vi "GCSArray_header_read.vi"(0 "GCSArray input string":string, 1 "Range":T2, 5 "error in (no error)":errorcluster) -> (14 "GCSArray Header":T1={"Identifier"="", "Version"=0, "Remark"="", "Dimension"=0, "Type"=enum."Matrix", "Separator"=0, "NData"=0, "NData%"=[], "Name%"=[], "Start%"=[], "End%"=[], "Delta%"=[], "SampleTime"=inf, "TransmittedUnit%"=[], "DisplayedUnit%"=[], "RatioNominator%"=[], "RatioDenominator%"=[]}, 19 "error out":errorcluster)   [LabVIEW 2026]
doc: "Transforms an Input string, limited to a specific character Range, into a GCSArray header.\n\nThe conversion of the textual representation of a GCSArray into the native format is performed using the LabVIEW regular expression engine. In case a header entry is not found its value is set to the default value, which is usually zero. The implemented functionality uses the GCS Array Data Format Description (Release 1.2.1, Date: 2010-09-27, PI document code: SM146E)."
uses:
  GCSArray_regex_range.ctl
  GCSArray_header.ctl
  GCSArray_header_action.ctl
  GCSArray_regex_selector.ctl
panel:
  in  "GCSArray_header":T1={"Identifier"="", "Version"=0, "Remark"="", "Dimension"=0, "Type"=enum."Matrix", "Separator"=0, "NData"=0, "NData%"=[], "Name%"=[], "Start%"=[], "End%"=[], "Delta%"=[], "SampleTime"=inf, "TransmittedUnit%"=[], "DisplayedUnit%"=[], "RatioNominator%"=[], "RatioDenominator%"=[]}
  # "Read a GCS Array string from, extract the header informations\naccording to the GCSArray definitions and return the\ncorresponding 'GCSArray Header' object."
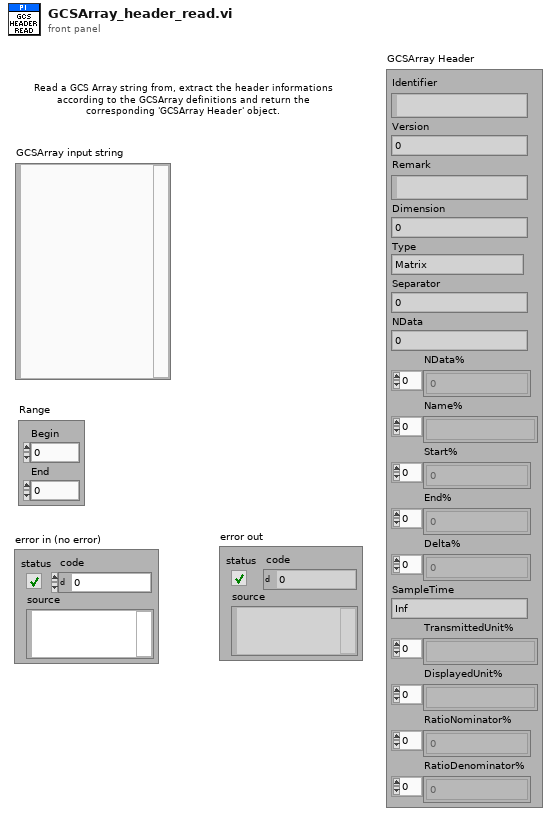
[diagram p1: front panel]
types:
  T1 = typedef "GCSArray_header.ctl" = cluster{"Identifier":string, "Version":i32, "Remark":string, "Dimension":i32, "Type":enum16{"Matrix", "Table"}, "Separator":u8, "NData":i32, "NData%":i32[], "Name%":string[], "Start%":dbl[], "End%":dbl[], "Delta%":dbl[], "SampleTime":dbl, "TransmittedUnit%":string[], "DisplayedUnit%":string[], "RatioNominator%":dbl[], "RatioDenominator%":dbl[]}
  T2 = typedef "GCSArray_regex_range.ctl" = cluster{"Begin":i32, "End":i32}
  T3 = typedef "GCSArray_regex_selector.ctl" = enum16{"GCS_ARRAY Block Full", "GCS_ARRAY Block ID", "GCS_ARRAY Block Header", "GCS_ARRAY Block Data", "GCS_ARRAY Identifier", "GCS_ARRAY Remark", "GCS_ARRAY Version", "GCS_ARRAY Dimension", "GCS_ARRAY Type", "GCS_ARRAY Separator", "GCS_ARRAY NData", "GCS_ARRAY NData%", "GCS_ARRAY NData% Keyword", "GCS_ARRAY Name%", "GCS_ARRAY Name% Keyword", "GCS_ARRAY Start%", "GCS_ARRAY Start% Keyword", "GCS_ARRAY End%", "GCS_ARRAY End% Keyword", "GCS_ARRAY Delta%", "GCS_ARRAY Delta% Keword", "GCS_ARRAY Sample Time", "GCS_ARRAY Unit of transmitted value%", "GCS_ARRAY Trans_Unit% Keyword", "GCS_ARRAY Trans_Unit% = RAW Keyword", "GCS_ARRAY Unit of displayed value%", "GCS_ARRAY Disp_Unit% Keyword", "GCS_ARRAY Nominator%", "GCS_ARRAY Ratio_Nom% Keyword", "GCS_ARRAY Denominator%", "GCS_ARRAY Ratio_Denom% Keyword", "GCS_ARRAY End of Header", "GCS_ARRAY Empty line of Header"}
  T4 = typedef "GCSArray_header_action.ctl" = enum16{"GCS_ARRAY_HEADER Identifier", "GCS_ARRAY_HEADER Version", "GCS_ARRAY_HEADER Remark", "GCS_ARRAY_HEADER Dimension", "GCS_ARRAY_HEADER Type", "GCS_ARRAY_HEADER Separator", "GCS_ARRAY_HEADER NData", "GCS_ARRAY_HEADER NData%", "GCS_ARRAY_HEADER Name%", "GCS_ARRAY_HEADER Start%", "GCS_ARRAY_HEADER End%", "GCS_ARRAY_HEADER Delta%", "GCS_ARRAY_HEADER Sample Time", "GCS_ARRAY_HEADER Unit of transmitted value%", "GCS_ARRAY_HEADER Unit of displayed unit%", "GCS_ARRAY_HEADER Nominator%", "GCS_ARRAY_HEADER Denominator%"}
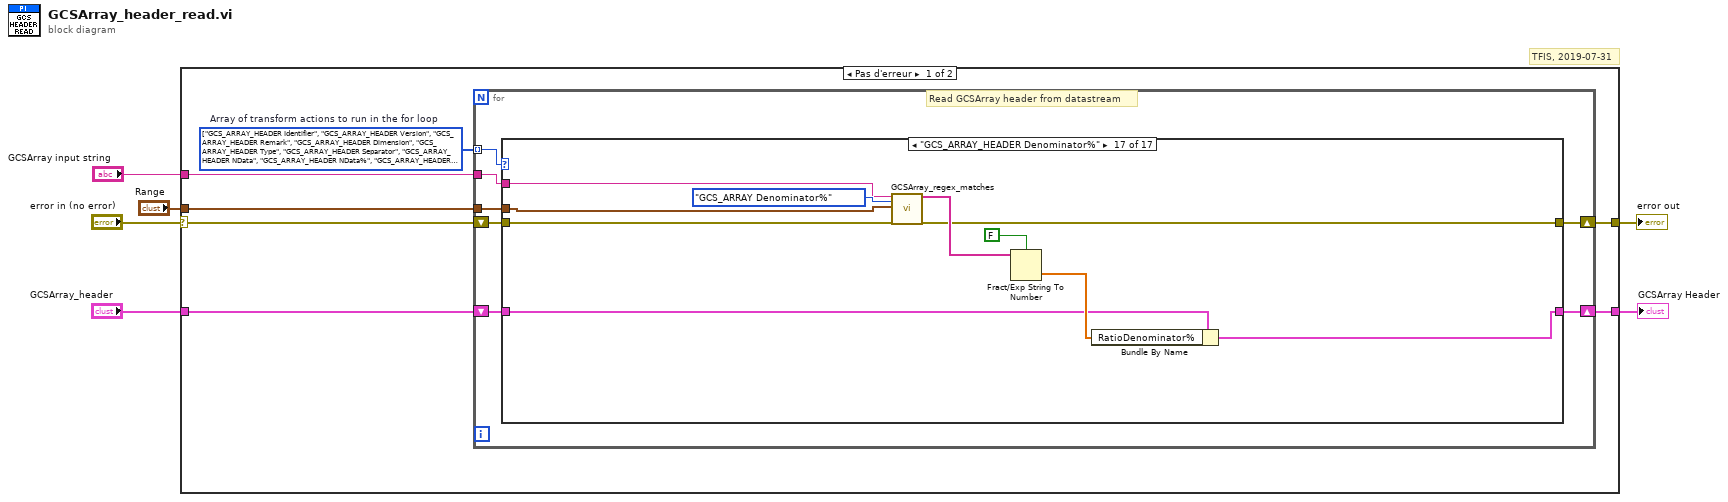
[diagram p0: block diagram]
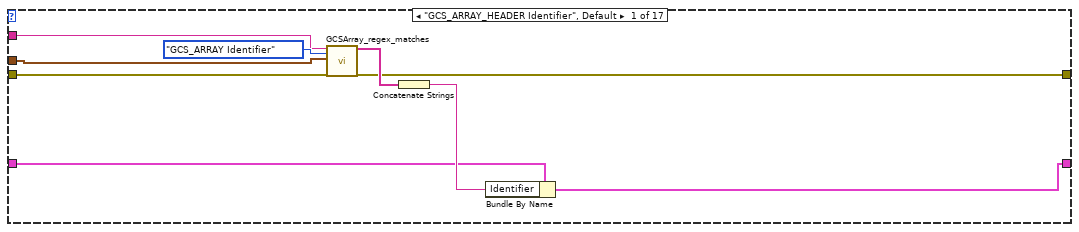
[diagram p2: hidden frame]
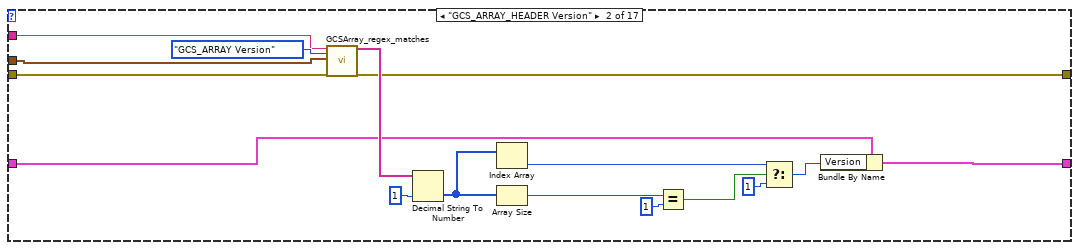
[diagram p3: hidden frame]
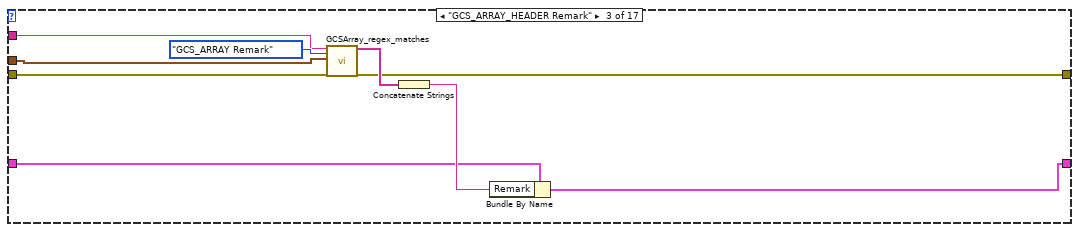
[diagram p4: hidden frame]
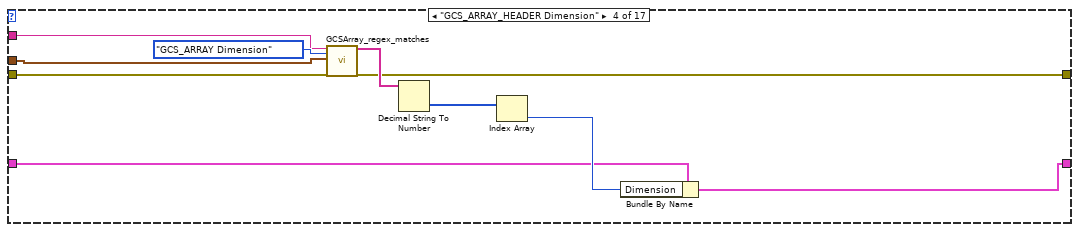
[diagram p5: hidden frame]
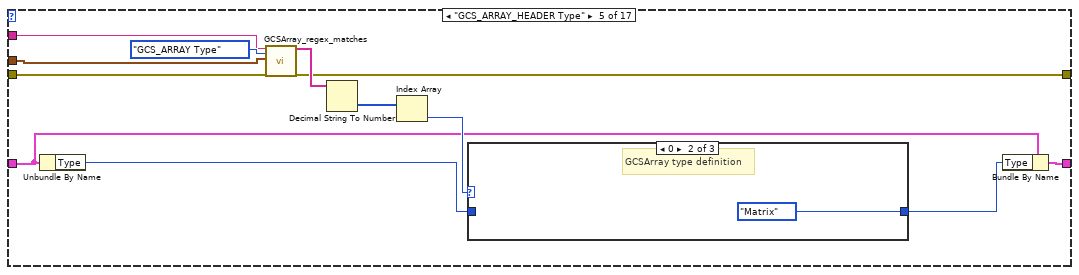
[diagram p6: hidden frame]
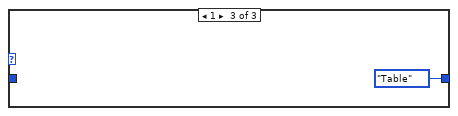
[diagram p8: hidden frame]
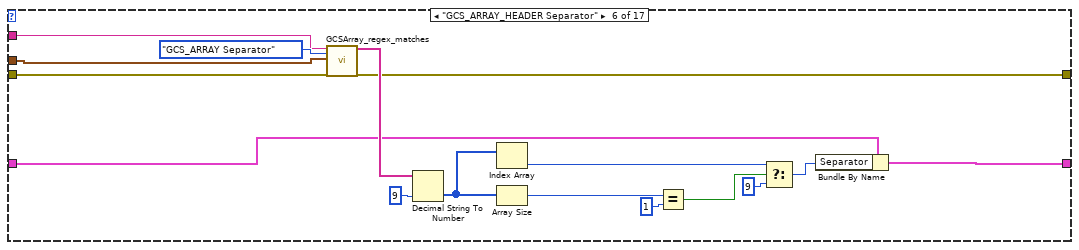
[diagram p9: hidden frame]
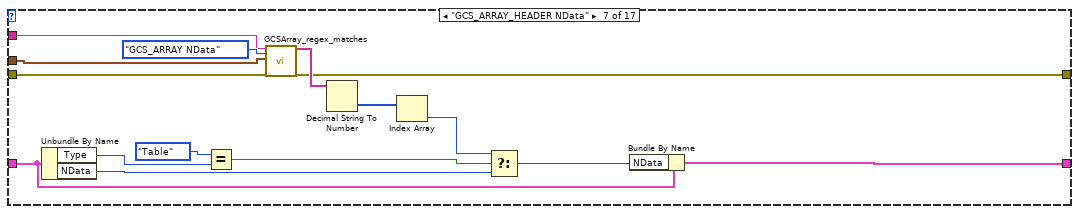
[diagram p10: hidden frame]
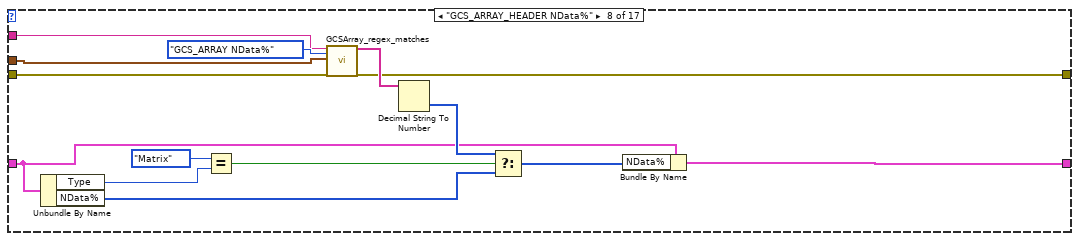
[diagram p11: hidden frame]
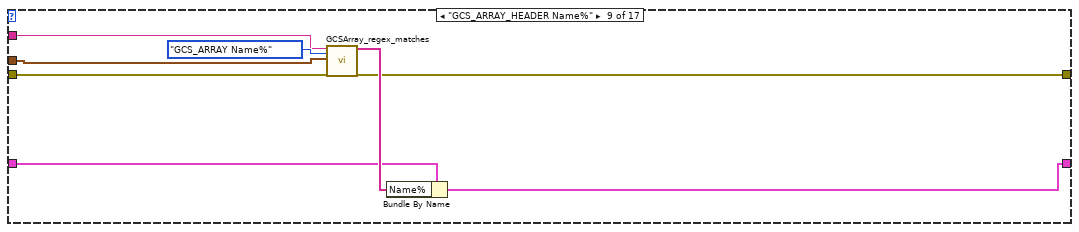
[diagram p12: hidden frame]
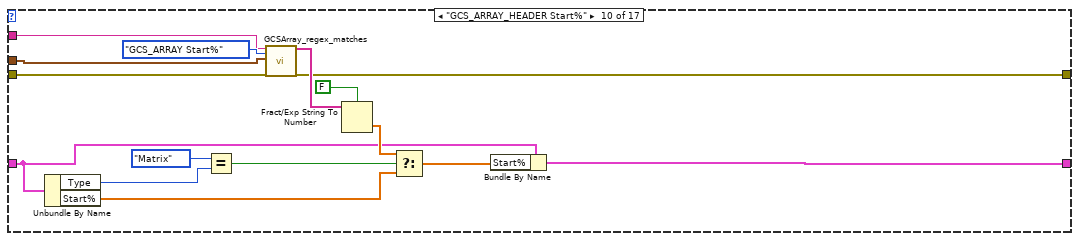
[diagram p13: hidden frame]
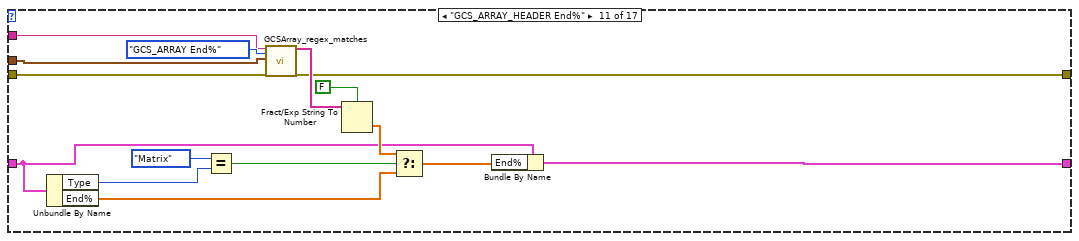
[diagram p14: hidden frame]
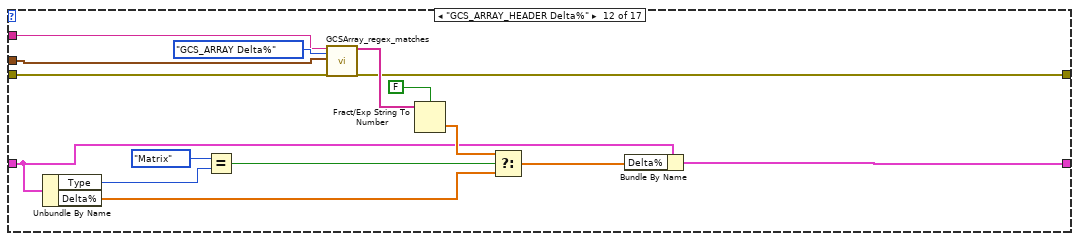
[diagram p15: hidden frame]
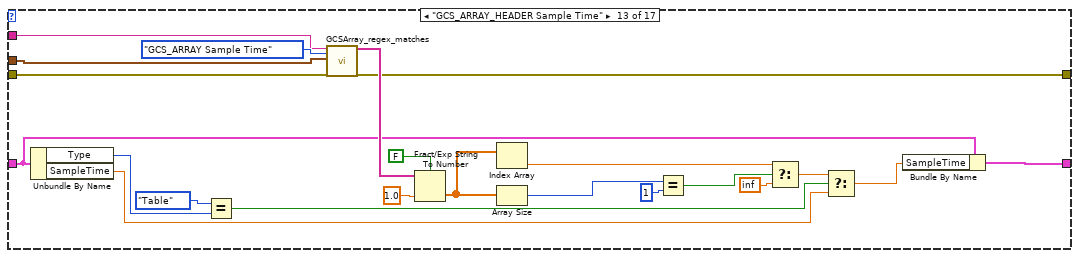
[diagram p16: hidden frame]
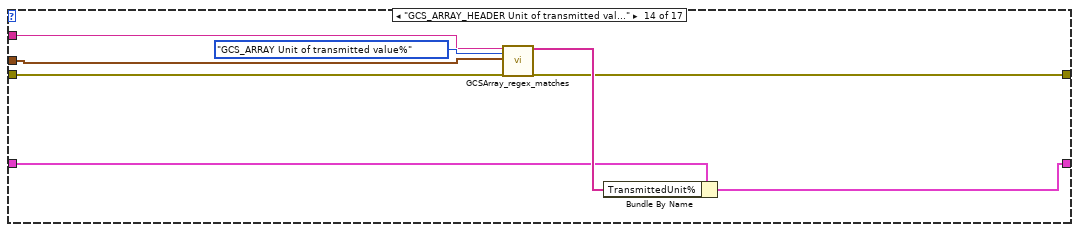
[diagram p17: hidden frame]
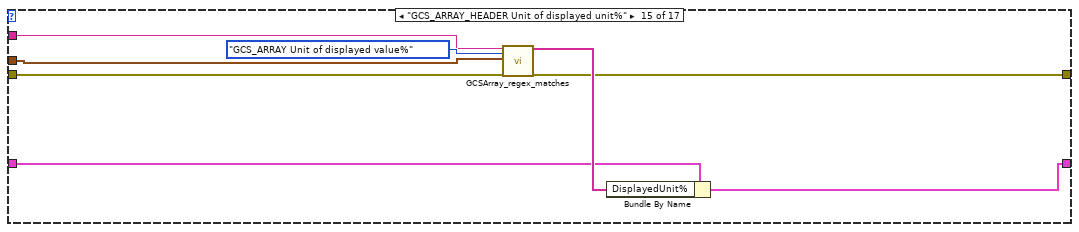
[diagram p18: hidden frame]
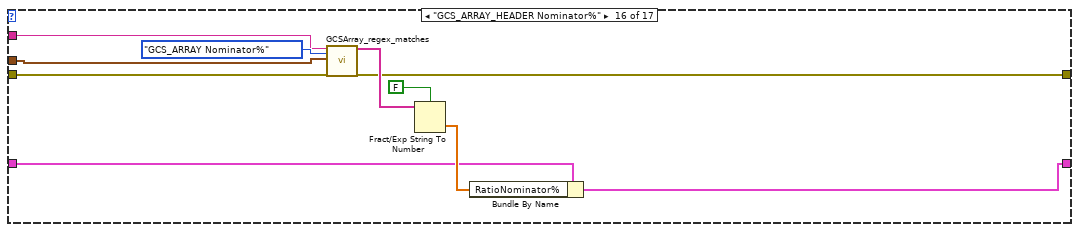
[diagram p19: hidden frame]
diagram:
  # "TFIS, 2019-07-31"
  n1 = case shown="Pas d'erreur" "error in (no error)" {
    selector: "error in (no error)" -> [w13 w237]
    tunnel: [w8 w237] -> w5
    tunnel: "GCSArray input string" -> [w11 _]
    tunnel: [w9 w236] -> w2
    tunnel: "Range" -> [w10 _]
    tunnel: "GCSArray_header" -> [w12 w236]
    frame No Error {
      w7 = T4[] [enum."GCS_ARRAY_HEADER Identifier", enum."GCS_ARRAY_HEADER Version", enum."GCS_ARRAY_HEADER Remark", enum."GCS_ARRAY_HEADER Dimension", enum."GCS_ARRAY_HEADER Type", enum."GCS_ARRAY_HEADER Separator", enum."GCS_ARRAY_HEADER NData", enum."GCS_ARRAY_HEADER NData%", enum."GCS_ARRAY_HEADER Name%", enum."GCS_ARRAY_HEADER Start%", enum."GCS_ARRAY_HEADER End%", enum."GCS_ARRAY_HEADER Delta%", enum."GCS_ARRAY_HEADER Sample Time", enum."GCS_ARRAY_HEADER Unit of transmitted value%", enum."GCS_ARRAY_HEADER Unit of displayed unit%", enum."GCS_ARRAY_HEADER Nominator%", enum."GCS_ARRAY_HEADER Denominator%"] items=["GCS_ARRAY_HEADER Identifier", "GCS_ARRAY_HEADER Version", "GCS_ARRAY_HEADER Remark", "GCS_ARRAY_HEADER Dimension", "GCS_ARRAY_HEADER Type", "GCS_ARRAY_HEADER Separator", "GCS_ARRAY_HEADER NData", "GCS_ARRAY_HEADER NData%", "GCS_ARRAY_HEADER Name%", "GCS_ARRAY_HEADER Start%", "GCS_ARRAY_HEADER End%", "GCS_ARRAY_HEADER Delta%", "GCS_ARRAY_HEADER Sample Time", "GCS_ARRAY_HEADER Unit of transmitted value%", "GCS_ARRAY_HEADER Unit of displayed unit%", "GCS_ARRAY_HEADER Nominator%", "GCS_ARRAY_HEADER Denominator%"]  # Array of transform actions to run in the for loop
      n2 = for {
        tunnel: w7 -> [w20] mode=indexing
        shift-right: [w18] -> w8
        shift-left: w13 -> [w19]
        shift-right: [w16] -> w9
        shift-left: w12 -> [w17]
        tunnel: w11 -> [w15]
        tunnel: w10 -> [w14]
        # "Read GCSArray header from datastream"
        n3 = case shown="\"GCS_ARRAY_HEADER Denominator%\"" w20 {
          tunnel: w19 -> [w26 w33 w51 w60 w68 w85 w99 w112 w130 w136 w153 w165 w183 w203 w212 w221 w226]
          tunnel: [w25 w32 w50 w59 w65 w82 w101 w116 w127 w137 w150 w168 w182 w200 w208 w218 w229] -> w18
          tunnel: w17 -> [w24 w31 w47 w56 w70 w80 w96 w114 w129 w135 w152 w166 w180 w202 w210 w222 w231]
          tunnel: [w23 w30 w46 w55 w69 w81 w100 w115 w128 w138 w151 w167 w181 w201 w209 w217 w230] -> w16
          tunnel: w15 -> [w22 w35 w49 w57 w66 w83 w97 w111 w126 w133 w148 w163 w178 w205 w213 w220 w228]
          tunnel: w14 -> [w21 w34 w48 w58 w67 w84 w98 w113 w125 w134 w149 w164 w179 w204 w211 w219 w227]
          frame "GCS_ARRAY_HEADER Identifier", Default {
            n4 = call "GCSArray_regex_matches.vi"("GCSArray input string"=w22, "Selector"=GCSArray_regex_selector."GCS_ARRAY Identifier", "Range"=w21, "error in (no error)"=w26) -> ("Matches"=w28:string[], "error out"=w25:errorcluster)  [unwired: 14 out]
            n5 = Concatenate Strings(w28) -> (w27:string)
            n6 = Bundle By Name(cluster=w24, "Identifier"=w27) -> (w23:T1)
          }
          frame "GCS_ARRAY_HEADER Version" {
            n7 = call "GCSArray_regex_matches.vi"("GCSArray input string"=w35, "Selector"=GCSArray_regex_selector."GCS_ARRAY Version", "Range"=w34, "error in (no error)"=w33) -> ("Matches"=w45:string[], "error out"=w32:errorcluster)  [unwired: 14 out]
            n8 = Decimal String To Number(string=w45, default (0L)=1 ("default (0 I32)")) -> (number=w40:i32[])  [unwired: 2 out]
            n9 = Index Array(array=w40) -> (element=w37:i32)  [unwired: 1 in]
            n10 = Array Size(array=w40) -> (size(s)=w42:i32)
            n11 = Equal?(x=w42, y=1) -> (x = y?=w38:bool)
            n12 = Select(t=w37, s=w38, f=1) -> (s? t:f=w36:i32)
            n13 = Bundle By Name(cluster=w31, "Version"=w36) -> (w30:T1)
          }
          frame "GCS_ARRAY_HEADER Remark" {
            n14 = call "GCSArray_regex_matches.vi"("GCSArray input string"=w49, "Selector"=GCSArray_regex_selector."GCS_ARRAY Remark", "Range"=w48, "error in (no error)"=w51) -> ("Matches"=w54:string[], "error out"=w50:errorcluster)  [unwired: 14 out]
            n15 = Concatenate Strings(w54) -> (w52:string)
            n16 = Bundle By Name(cluster=w47, "Remark"=w52) -> (w46:T1)
          }
          frame "GCS_ARRAY_HEADER Dimension" {
            n17 = call "GCSArray_regex_matches.vi"("GCSArray input string"=w57, "Selector"=GCSArray_regex_selector."GCS_ARRAY Dimension", "Range"=w58, "error in (no error)"=w60) -> ("Matches"=w63:string[], "error out"=w59:errorcluster)  [unwired: 14 out]
            n18 = Decimal String To Number(string=w63) -> (number=w64:i32[])  [unwired: 3 out]
            n19 = Index Array(array=w64) -> (element=w61:i32)  [unwired: 1 in]
            n20 = Bundle By Name(cluster=w56, "Dimension"=w61) -> (w55:T1)
          }
          frame "GCS_ARRAY_HEADER Type" {
            n21 = Unbundle By Name(w70) -> ("Type"=w71:enum16{"Matrix", "Table"})
            n22 = call "GCSArray_regex_matches.vi"("GCSArray input string"=w66, "Selector"=GCSArray_regex_selector."GCS_ARRAY Type", "Range"=w67, "error in (no error)"=w68) -> ("Matches"=w75:string[], "error out"=w65:errorcluster)  [unwired: 14 out]
            n23 = Decimal String To Number(string=w75) -> (number=w76:i32[])  [unwired: 3 out]
            n24 = Index Array(array=w76) -> (element=w73:i32)  [unwired: 1 in]
            n25 = case shown="0" w73 {
              tunnel: [w77 enum16{"Matrix", "Table"}."Matrix" ("Type") enum16{"Matrix", "Table"}."Table" ("Type")] -> w72
              tunnel: w71 -> [w77 _ _]
              frame -1, Default {
              }
              frame 0 {
                # "GCSArray type definition"
              }
              frame 1 {
              }
            }
            n26 = Bundle By Name(cluster=w70, "Type"=w72) -> (w69:T1)
          }
          frame "GCS_ARRAY_HEADER Separator" {
            n27 = call "GCSArray_regex_matches.vi"("GCSArray input string"=w83, "Selector"=GCSArray_regex_selector."GCS_ARRAY Separator", "Range"=w84, "error in (no error)"=w85) -> ("Matches"=w95:string[], "error out"=w82:errorcluster)  [unwired: 14 out]
            n28 = Decimal String To Number(string=w95, default (0L)=9 ("default (0 I32)")) -> (number=w92:i32[])  [unwired: 2 out]
            n29 = Index Array(array=w92) -> (element=w88:i32)  [unwired: 1 in]
            n30 = Array Size(array=w92) -> (size(s)=w91:i32)
            n31 = Equal?(x=w91, y=1) -> (x = y?=w89:bool)
            n32 = Select(t=w88, s=w89, f=9) -> (s? t:f=w86:i32)
            n33 = Bundle By Name(cluster=w80, "Separator"=w86) -> (w81:T1)
          }
          frame "GCS_ARRAY_HEADER NData" {
            n34 = Unbundle By Name(w96) -> ("Type"=w107:enum16{"Matrix", "Table"}, "NData"=w103:i32)
            n35 = Equal?(x=enum16{"Matrix", "Table"}."Table" ("y"), y=w107) -> (x = y?=w105:bool)
            n36 = call "GCSArray_regex_matches.vi"("GCSArray input string"=w97, "Selector"=GCSArray_regex_selector."GCS_ARRAY NData", "Range"=w98, "error in (no error)"=w99) -> ("Matches"=w109:string[], "error out"=w101:errorcluster)  [unwired: 14 out]
            n37 = Decimal String To Number(string=w109) -> (number=w110:i32[])  [unwired: 3 out]
            n38 = Index Array(array=w110) -> (element=w104:i32)  [unwired: 1 in]
            n39 = Select(t=w104, s=w105, f=w103) -> (s? t:f=w102:i32)
            n40 = Bundle By Name(cluster=w96, "NData"=w102) -> (w100:T1)
          }
          frame "GCS_ARRAY_HEADER NData%" {
            n41 = Unbundle By Name(w114) -> ("Type"=w122:enum16{"Matrix", "Table"}, "NData%"=w119:i32[])
            n42 = Equal?(x=enum16{"Matrix", "Table"}."Matrix" ("y"), y=w122) -> (x = y?=w120:bool)
            n43 = call "GCSArray_regex_matches.vi"("GCSArray input string"=w111, "Selector"=GCSArray_regex_selector."GCS_ARRAY NData%", "Range"=w113, "error in (no error)"=w112) -> ("Matches"=w124:string[], "error out"=w116:errorcluster)  [unwired: 14 out]
            n44 = Decimal String To Number(string=w124) -> (number=w118:i32[])  [unwired: 3 out]
            n45 = Select(t=w118, s=w120, f=w119) -> (s? t:f=w117:i32[])
            n46 = Bundle By Name(cluster=w114, "NData%"=w117) -> (w115:T1)
          }
          frame "GCS_ARRAY_HEADER Name%" {
            n47 = call "GCSArray_regex_matches.vi"("GCSArray input string"=w126, "Selector"=GCSArray_regex_selector."GCS_ARRAY Name%", "Range"=w125, "error in (no error)"=w130) -> ("Matches"=w131:string[], "error out"=w127:errorcluster)  [unwired: 14 out]
            n48 = Bundle By Name(cluster=w129, "Name%"=w131) -> (w128:T1)
          }
          frame "GCS_ARRAY_HEADER Start%" {
            n49 = Unbundle By Name(w135) -> ("Type"=w145:enum16{"Matrix", "Table"}, "Start%"=w140:dbl[])
            n50 = Equal?(x=enum16{"Matrix", "Table"}."Matrix" ("y"), y=w145) -> (x = y?=w143:bool)
            n51 = call "GCSArray_regex_matches.vi"("GCSArray input string"=w133, "Selector"=GCSArray_regex_selector."GCS_ARRAY Start%", "Range"=w134, "error in (no error)"=w136) -> ("Matches"=w146:string[], "error out"=w137:errorcluster)  [unwired: 14 out]
            n52 = Fract/Exp String To Number(use system decimal point (T)=FALSE, string=w146) -> (number=w142:dbl[])  [unwired: 3 out]
            n53 = Select(t=w142, s=w143, f=w140) -> (s? t:f=w141:dbl[])
            n54 = Bundle By Name(cluster=w135, "Start%"=w141) -> (w138:T1)
          }
          frame "GCS_ARRAY_HEADER End%" {
            n55 = Unbundle By Name(w152) -> ("Type"=w160:enum16{"Matrix", "Table"}, "End%"=w155:dbl[])
            n56 = Equal?(x=enum16{"Matrix", "Table"}."Matrix" ("y"), y=w160) -> (x = y?=w158:bool)
            n57 = call "GCSArray_regex_matches.vi"("GCSArray input string"=w148, "Selector"=GCSArray_regex_selector."GCS_ARRAY End%", "Range"=w149, "error in (no error)"=w153) -> ("Matches"=w161:string[], "error out"=w150:errorcluster)  [unwired: 14 out]
            n58 = Fract/Exp String To Number(use system decimal point (T)=FALSE, string=w161) -> (number=w157:dbl[])  [unwired: 3 out]
            n59 = Select(t=w157, s=w158, f=w155) -> (s? t:f=w156:dbl[])
            n60 = Bundle By Name(cluster=w152, "End%"=w156) -> (w151:T1)
          }
          frame "GCS_ARRAY_HEADER Delta%" {
            n61 = Unbundle By Name(w166) -> ("Type"=w175:enum16{"Matrix", "Table"}, "Delta%"=w170:dbl[])
            n62 = Equal?(x=enum16{"Matrix", "Table"}."Matrix" ("y"), y=w175) -> (x = y?=w173:bool)
            n63 = call "GCSArray_regex_matches.vi"("GCSArray input string"=w163, "Selector"=GCSArray_regex_selector."GCS_ARRAY Delta%", "Range"=w164, "error in (no error)"=w165) -> ("Matches"=w176:string[], "error out"=w168:errorcluster)  [unwired: 14 out]
            n64 = Fract/Exp String To Number(use system decimal point (T)=FALSE, string=w176) -> (number=w172:dbl[])  [unwired: 3 out]
            n65 = Select(t=w172, s=w173, f=w170) -> (s? t:f=w171:dbl[])
            n66 = Bundle By Name(cluster=w166, "Delta%"=w171) -> (w167:T1)
          }
          frame "GCS_ARRAY_HEADER Sample Time" {
            n67 = Unbundle By Name(w180) -> ("Type"=w196:enum16{"Matrix", "Table"}, "SampleTime"=w193:dbl)
            n68 = Equal?(x=enum16{"Matrix", "Table"}."Table" ("y"), y=w196) -> (x = y?=w195:bool)
            n69 = call "GCSArray_regex_matches.vi"("GCSArray input string"=w178, "Selector"=GCSArray_regex_selector."GCS_ARRAY Sample Time", "Range"=w179, "error in (no error)"=w183) -> ("Matches"=w198:string[], "error out"=w182:errorcluster)  [unwired: 14 out]
            n70 = Fract/Exp String To Number(use system decimal point (T)=FALSE, string=w198, default (0 dbl)=1.0 ("default (0 DBL)")) -> (number=w190:dbl[])  [unwired: 2 out]
            n71 = Index Array(array=w190) -> (element=w186:dbl)  [unwired: 1 in]
            n72 = Array Size(array=w190) -> (size(s)=w189:i32)
            n73 = Equal?(x=w189, y=1) -> (x = y?=w187:bool)
            n74 = Select(t=w186, s=w187, f=inf) -> (s? t:f=w185:dbl)
            n75 = Select(t=w185, s=w195, f=w193) -> (s? t:f=w194:dbl)
            n76 = Bundle By Name(cluster=w180, "SampleTime"=w194) -> (w181:T1)
          }
          frame "GCS_ARRAY_HEADER Unit of transmitted value%" {
            n77 = call "GCSArray_regex_matches.vi"("GCSArray input string"=w205, "Selector"=GCSArray_regex_selector."GCS_ARRAY Unit of transmitted value%", "Range"=w204, "error in (no error)"=w203) -> ("Matches"=w206:string[], "error out"=w200:errorcluster)  [unwired: 14 out]
            n78 = Bundle By Name(cluster=w202, "TransmittedUnit%"=w206) -> (w201:T1)
          }
          frame "GCS_ARRAY_HEADER Unit of displayed unit%" {
            n79 = call "GCSArray_regex_matches.vi"("GCSArray input string"=w213, "Selector"=GCSArray_regex_selector."GCS_ARRAY Unit of displayed value%", "Range"=w211, "error in (no error)"=w212) -> ("Matches"=w214:string[], "error out"=w208:errorcluster)  [unwired: 14 out]
            n80 = Bundle By Name(cluster=w210, "DisplayedUnit%"=w214) -> (w209:T1)
          }
          frame "GCS_ARRAY_HEADER Nominator%" {
            n81 = call "GCSArray_regex_matches.vi"("GCSArray input string"=w220, "Selector"=GCSArray_regex_selector."GCS_ARRAY Nominator%", "Range"=w219, "error in (no error)"=w221) -> ("Matches"=w224:string[], "error out"=w218:errorcluster)  [unwired: 14 out]
            n82 = Fract/Exp String To Number(use system decimal point (T)=FALSE, string=w224) -> (number=w223:dbl[])  [unwired: 3 out]
            n83 = Bundle By Name(cluster=w222, "RatioNominator%"=w223) -> (w217:T1)
          }
          frame "GCS_ARRAY_HEADER Denominator%" {
            n84 = call "GCSArray_regex_matches.vi"("GCSArray input string"=w228, "Selector"=GCSArray_regex_selector."GCS_ARRAY Denominator%", "Range"=w227, "error in (no error)"=w226) -> ("Matches"=w234:string[], "error out"=w229:errorcluster)  [unwired: 14 out]
            n85 = Fract/Exp String To Number(use system decimal point (T)=FALSE, string=w234) -> (number=w233:dbl[])  [unwired: 3 out]
            n86 = Bundle By Name(cluster=w231, "RatioDenominator%"=w233) -> (w230:T1)
          }
        }
      }
    }
    frame Error {
    }
  }
  "error out" <- w5
  "GCSArray Header" <- w2
